vi "SimpleOscillate.vi"() -> ()   [LabVIEW 2010]
uses:
  Motion/EnableSingle.vi
panel:
  in  "taskId":i32(ring)=1 items=["TLibrary", "T01", "T02", "T03", "T04", "T05", "T06", "T07", "T08", "T09", "T10", "T11", "T12", "T13", "T14", "T15", "T16", "T17", "T18", "T19", "T20", "T21", "T22", "T23", "T24", "T25", "T26", "T27", "T28", "T29", "T30", "T31"]
  in  "axis name":string="X"
  in  "Disconnect After?":bool
  in  "NumFreqs":i32=2
  in  "Cycles":i32=2
  in  "Distance":dbl=50.0
  in  "Frequency":dbl=1.0
  out "error out":errorcluster
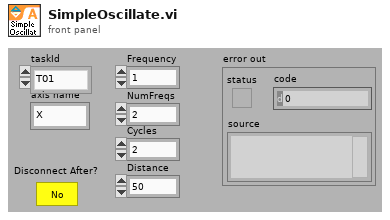
[diagram p1: front panel]
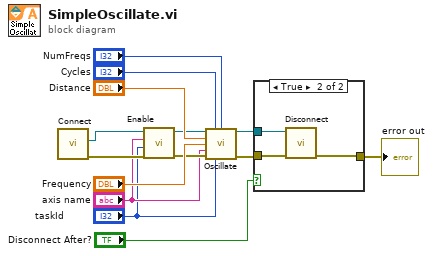
[diagram p0: block diagram]
diagram:
  n1 = call "Connect.vi"() -> ("error out"=w5:errorcluster, "controller"=w3:refnum<k24>)  [unwired: 10 in]
  n2 = call-poly "Enable.vi"("error in (no error)"=w5, "taskId"="taskId", "axis name"="axis name", "controller in"=w3) -> ("error out"=w4:errorcluster, "controller out"=w6:refnum<k24>)  [unwired: 6 in]
  n3 = call "Oscillate.vi"("controller in"=w6, "Cycles"="Cycles", "NumFreqs"="NumFreqs", "Distance"="Distance", "Frequency"="Frequency", "axis name"="axis name", "error in (no error)"=w4, "taskId"="taskId") -> ("controller out"=w7:refnum<k24>, "error out"=w13:errorcluster)  [unwired: 6 in]
  n4 = case shown="True" "Disconnect After?" {
    tunnel: [w15 w18] -> w14
    tunnel: w13 -> [w15 w17]
    tunnel: w7 -> [_ w16]
    frame False {
    }
    frame True {
      n5 = call "Disconnect.vi"("error in (no error)"=w17, "controller"=w16) -> ("error out"=w18:errorcluster)  [unwired: 9 in]
    }
  }
  "error out" <- w14
